vi "Open.vi"(8 "error in (no error)":errorcluster, 10 "Device Index":u32, 11 "RTL-SDR in":refnum<class "RTL-SDR.lvclass">) -> (0 "error out":errorcluster, 1 "function return":i32, 3 "RTL-SDR out":refnum<class "RTL-SDR.lvclass">)   [LabVIEW 2015, in "RTL-SDR.lvclass"]
doc: "Created IvanLis by LabVIEW Portal\nProfile: http://labviewportal.org/memberlist.php?mode=viewprofile&u=987\neMail: IvanLisanov@gMail.com\nTelegram: https://t.me/IvanLis"
uses:
  RTL-SDR.lvclass
  RTL-SDR.lvclass/RTL-SDR.ctl
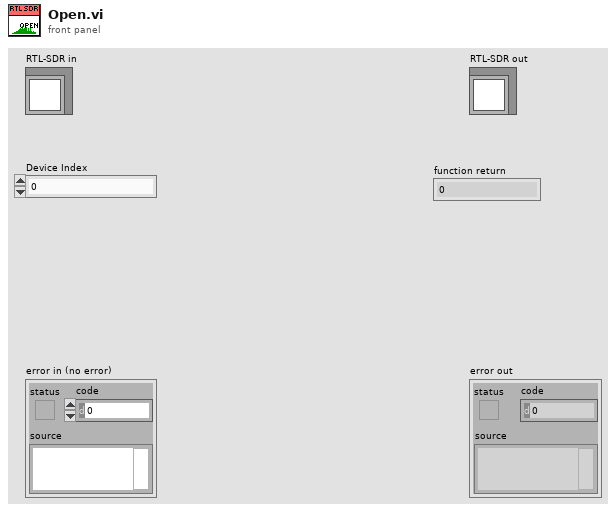
[diagram p1: front panel]
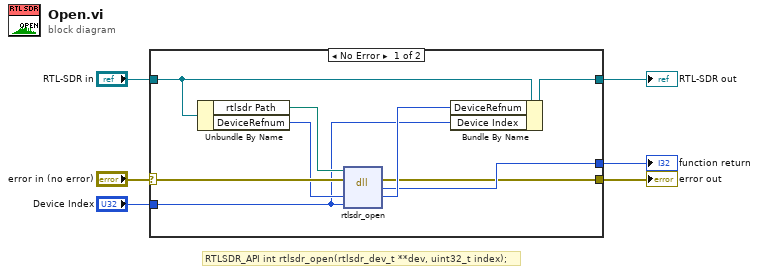
[diagram p0: block diagram]
diagram:
  # "RTLSDR_API int rtlsdr_open(rtlsdr_dev_t **dev, uint32_t index);"
  n1 = case shown="No Error" "error in (no error)" {
    selector: "error in (no error)" -> [w14 w17]
    tunnel: [w7 w17] -> w5
    tunnel: [w11 w16] -> w3
    tunnel: "RTL-SDR in" -> [w15 w16]
    tunnel: [w8 _] -> w2
    tunnel: "Device Index" -> [w9 _]
    frame No Error {
      n2 = Unbundle By Name(w15) -> ("rtlsdr Path"=w12:path, "DeviceRefnum"=w13:u64)
      n3 = dll-call lib="C:/Users/Ivan/Desktop/D-23-09-24 (RTL-SDR)/Project (Pelleng-SDR)/rtlsdr/dll/rtlsdr.*" fn="rtlsdr_open"(path in=w12, error in=w14, "DeviceRefnum"=w13, "index"=w9) -> (error out=w7:errorcluster, "return type"=w8:i32, "DeviceRefnum"=w10:u64)  [unwired: 2 in, 1 out]
      n4 = Bundle By Name(cluster=w15, "DeviceRefnum"=w10, "Device Index"=w9) -> (w11:refnum<class "RTL-SDR.lvclass">)
    }
    frame Error {
    }
  }
  "error out" <- w5
  "RTL-SDR out" <- w3
  "function return" <- w2
